vi "Current draw detection.vi"(9 "Time to Free spin (s)":dbl, 10 "OverCurrent":dbl, 11 "Current":dbl) -> (3 "Normal?":bool)   [LabVIEW 2015]
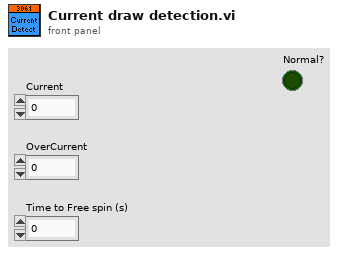
[diagram p1: front panel]
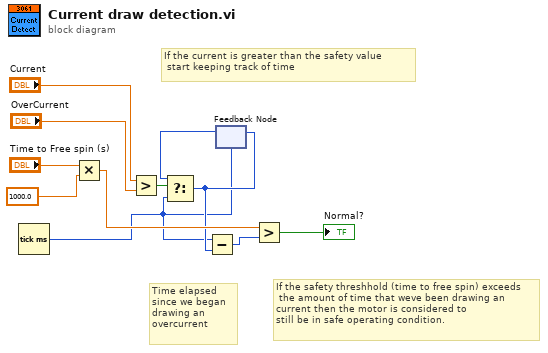
[diagram p0: block diagram]
diagram:
  # "Time elapsed\nsince we began \ndrawing an \novercurrent"
  # "If the safety threshhold (time to free spin) exceeds\n the amount of time that weve been drawing an \ncurrent then the motor is considered to\nstill be in safe operating condition."
  # "If the current is greater than the safety value\n start keeping track of time"
  n1 = Tick Count (ms)() -> (millisecond timer value=w2:u32)
  n2 = Multiply(x="Time to Free spin (s)", y=1000.0) -> (x*y=w7:dbl)
  n3 = Greater?(x="Current", y="OverCurrent") -> (0:w9:bool)
  n4 = feedback #1(w2) -> (w5:u32)
  n5 = Select(t=w5, s=w9, f=w2) -> (s? t:f=w3:u32)
  n6 = Subtract(x=w2, y=w3) -> (x-y=w4:u32)
  n7 = feedback-in #1(w3) -> ()
  n8 = Greater?(x=w7, y=w4) -> (0:→"Normal?":bool)
